vi "Configure RF Phase.vi"(6 "Phase Wrapping Degrees (180)":i32=180, 8 "error in (no error)":errorcluster, 9 "Enable Phase Wrapping (T: Enable)":bool=TRUE, 10 "Reference Degrees (0)":i32, 11 "VISA resource name":refnum<visa-resource-name>) -> (0 "error out":errorcluster, 3 "VISA resource name out":refnum<visa-resource-name>)   [LabVIEW 2016, in "Tektronix DPO MSO 2000 4000 Series.lvlib"]
doc: "Configures the phase on the RF Phase time domain channel.\n\n<B>Note:</B>\nOnly valid on <B>MDO 4000B and MDO 4000C</B> series instruments."
uses:
  Tektronix DPO MSO 2000 4000 Series.lvlib
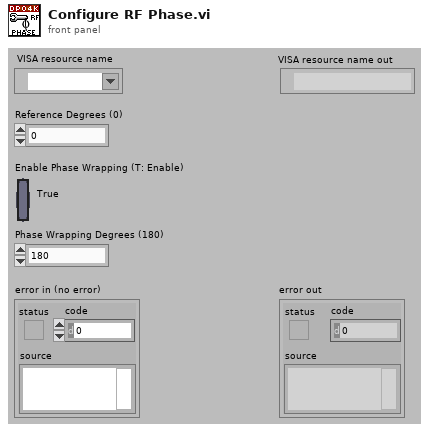
[diagram p1: front panel]
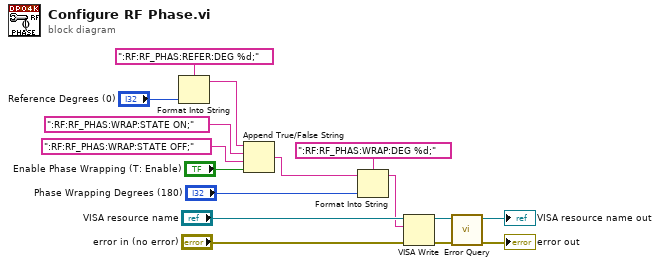
[diagram p0: block diagram]
diagram:
  n1 = Format Into String(format string=":RF:RF_PHAS:REFER:DEG %d;", "Reference Degrees (0)") -> (resulting string=w3:string)  [unwired: 2 in, 1 out]
  n2 = Append True/False String(1:"Enable Phase Wrapping (T: Enable)", 2:":RF:RF_PHAS:WRAP:STATE OFF;" ("false string"), 3:":RF:RF_PHAS:WRAP:STATE ON;" ("false string"), 4:w3) -> (0:w7:string)
  n3 = Format Into String(format string=":RF:RF_PHAS:WRAP:DEG %d;", initial string=w7, "Phase Wrapping Degrees (180)") -> (resulting string=w8:string)  [unwired: 1 in, 1 out]
  n4 = VISA Write(VISA resource name="VISA resource name", write buffer=w8, error in (no error)="error in (no error)") -> (VISA resource name out=w11:refnum<visa-resource-name>, error out=w14:errorcluster)  [unwired: 1 out]
  n5 = call "Error Query.vi"("error in (no error)"=w14, "VISA resource name"=w11) -> ("error out"=→"error out":errorcluster, "VISA resource name out"=→"VISA resource name out":refnum<visa-resource-name>)  [unwired: 6 in, 2 out]
